vi "SerialFrameProtocol_1_test.vi"() -> ()   [LabVIEW 2015]
uses:
  <vilib>/Instr/_visa.llb/VISA Flush IO Buffer Mask.ctl
  <vilib>/Instr/_visa.llb/VISA Set IO Buffer Mask.ctl
  <vilib>/Instr/_visa.llb/VISA Configure Serial Port (Instr).vi
panel:
  in  "VISA resource name":refnum<visa-resource-name>="COM6"
  out "buffer, NORMAL == read buffer unstuffing, NORMAL":bool
  out "size(s)":i32
  out "size(s)":i32
  out "Receiv Array":u8[](array[numeric])
  out "Send Array":u8[](array[numeric])
  out "Data2 (U16)":u16[](array[numeric])
  out "size(Data2)":i32
  out "size(Data1)":i32
  out "Data1 (I32)":i32[](array[numeric])
  out "B0":cluster{"iVal":i32, "fVal":sgl}
  out "buffer, HEX":string
  out "buffer, NORMAL":string
  out "buffer stuffing, HEX":string
  in  "Clear log":bool
  in  "CA":bool
  out "log":string
  in  "CL":bool
  in  "CZ":bool
  out "VISA Read counter":i32
  out "error IO":errorcluster
  out "VISA Read no error counter":i32
  in  "CN":bool
  in  "CY":bool
  in  "CB":bool
  out "CX Send array == AX read array":bool
  out "read buffer unstuffing, HEX":string
  out "read buffer unstuffing, NORMAL":string
  out "buffer stuffing, NORMAL":string
  out "read buffer RAW, HEX":string
  in  "stop":bool
  out "Counter":i32
  out "read buffer RAW, NORMAL":string="\n"
  in  "CX Send rand array":bool
  # "Serial Frame Protocol Test"
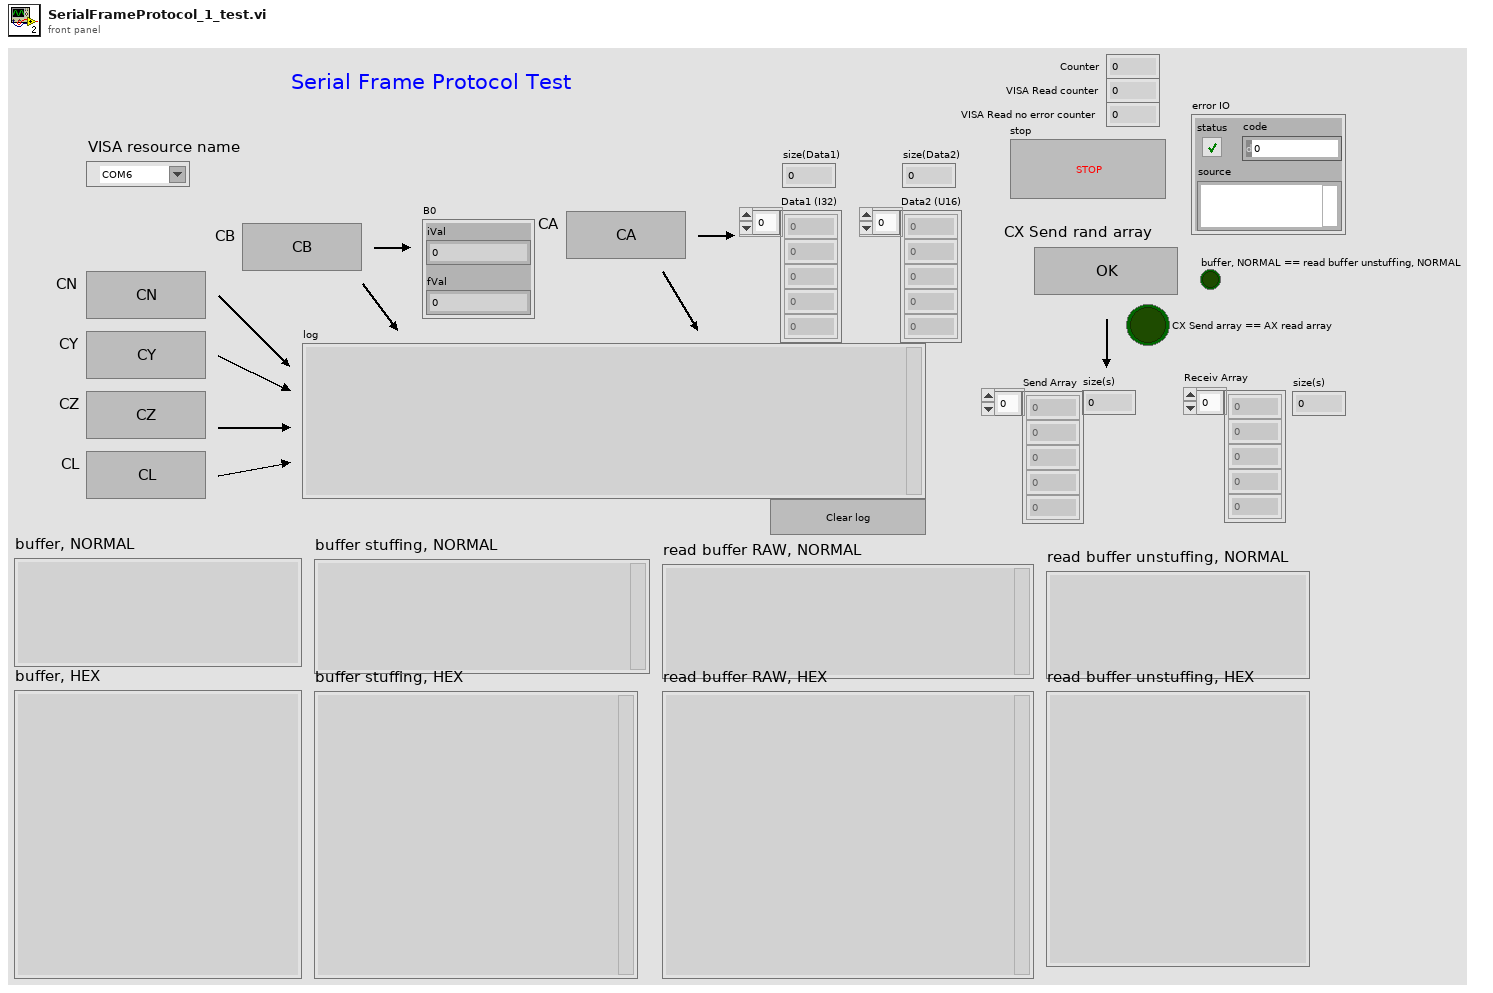
[diagram p1: front panel]
types:
  T1 = typedef "VISA Set IO Buffer Mask.ctl" = u16
  T2 = typedef "VISA Flush IO Buffer Mask.ctl" = u16
  T3 = enum16{"big-endian, network order", "native, host order", "little-endian"}
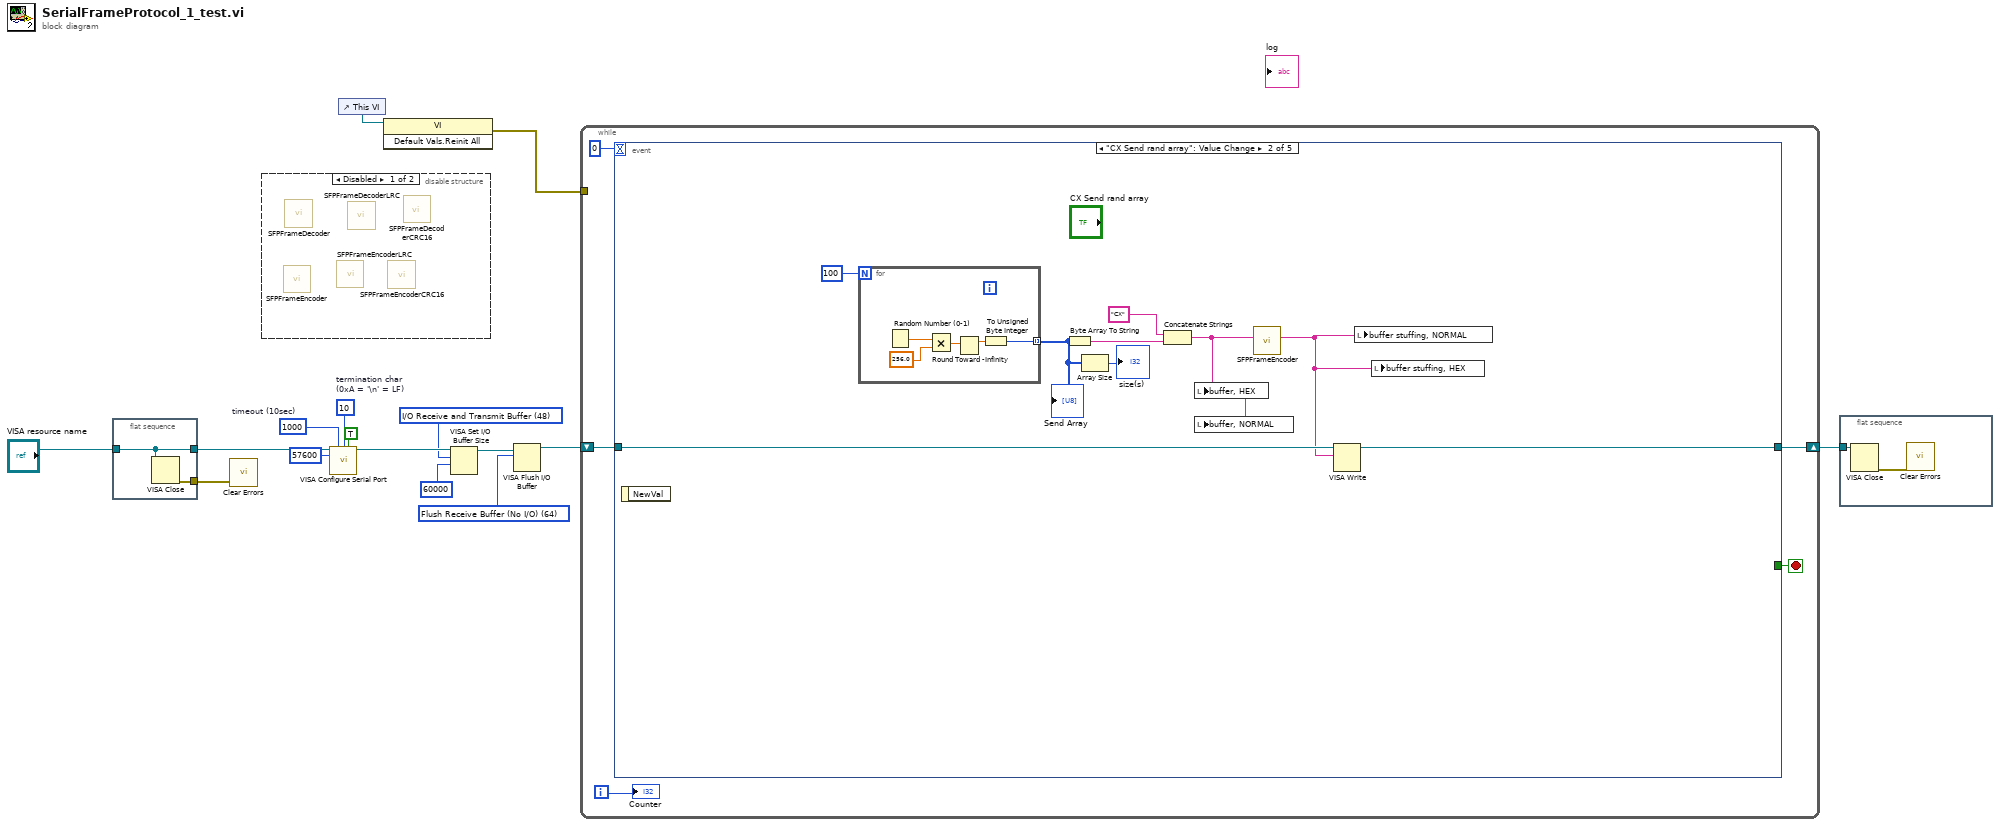
[diagram p0: block diagram]
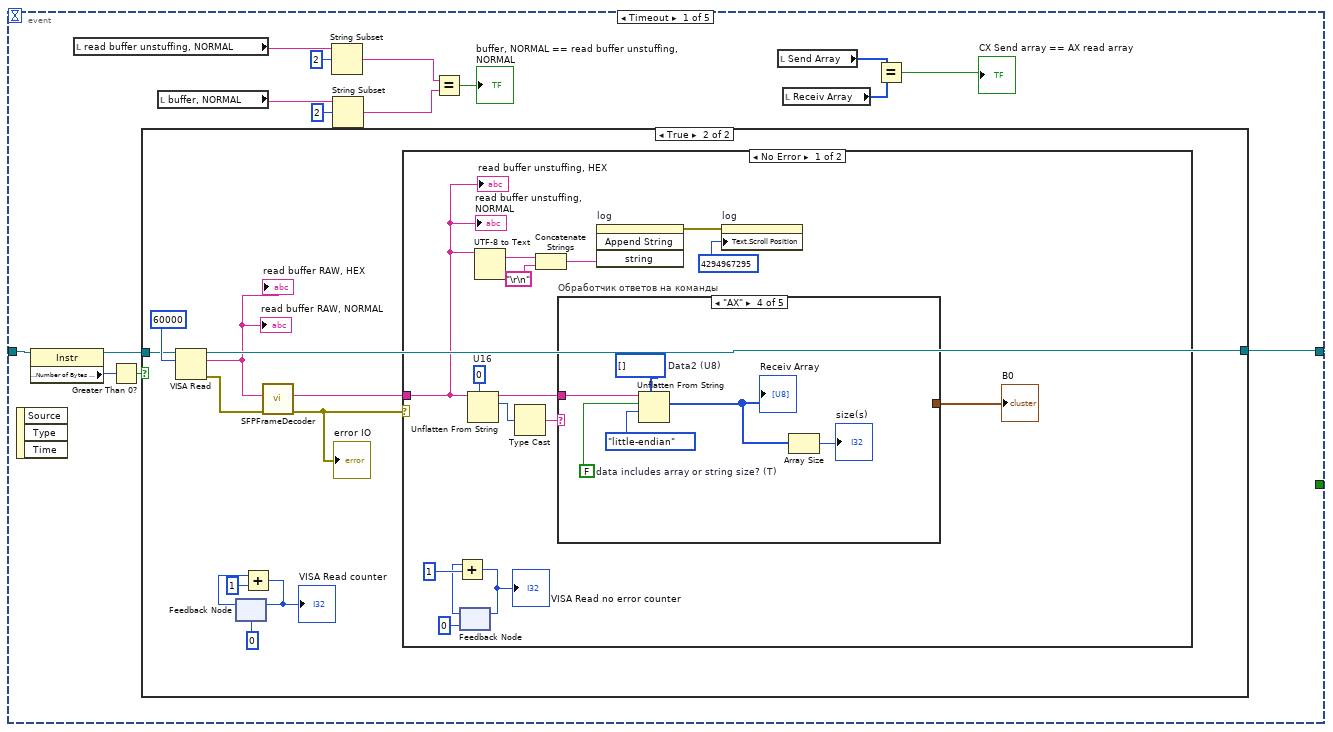
[diagram p2: hidden frame]
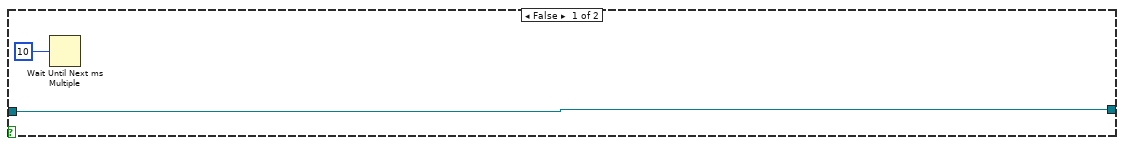
[diagram p3: hidden frame]
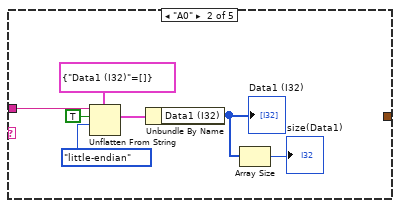
[diagram p5: hidden frame]
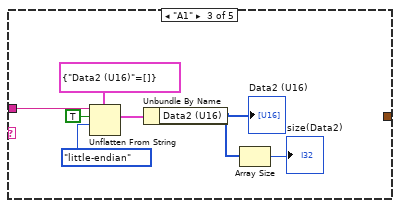
[diagram p6: hidden frame]
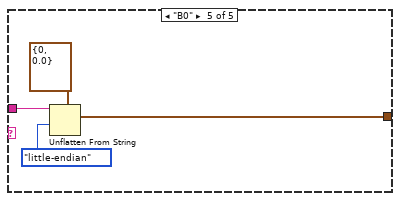
[diagram p7: hidden frame]
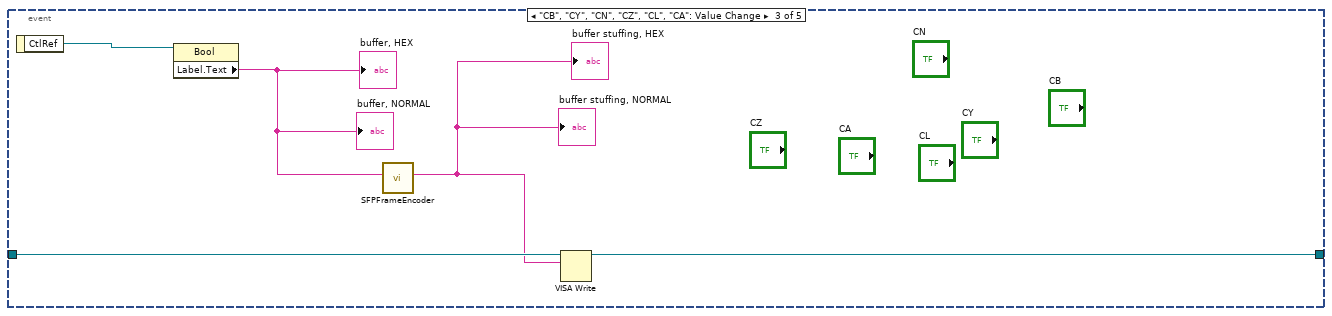
[diagram p9: hidden frame]
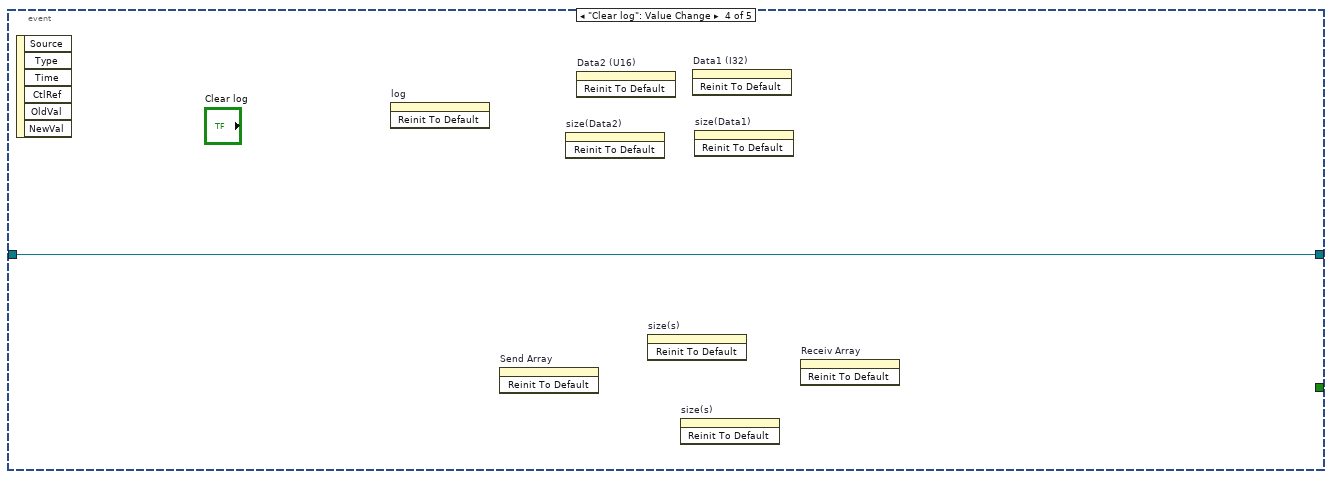
[diagram p10: hidden frame]
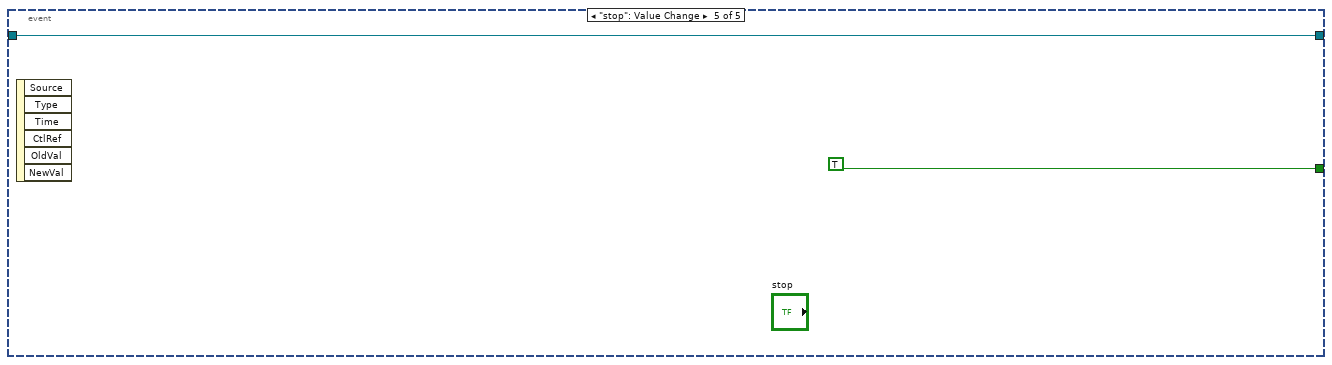
[diagram p11: hidden frame]
diagram:
  w3 = T1 48 items=["I/O Receive Buffer"=16, "I/O Transmit Buffer"=32, "I/O Receive and Transmit Buffer"=48] ("Mask")
  w5 = T2 64 items=["Flush Receive Buffer"=16, "Write Transmit Buffer to Device"=32, "Flush Receive Buffer (No I/O)"=64, "Flush Transmit Buffer"=128] ("Mask")
  w11 = u8 10  # termination char (0xA = '\n' = LF)
  w13 = u32 1000  # timeout (10sec)
  n1 = flat-sequence {
    tunnel: "VISA resource name" -> [w18]
    tunnel: [w18] -> w9
    tunnel: [w17] -> w16
    frame #0 {
      n2 = VISA Close(VISA resource name=w18) -> (error out=w17:errorcluster)  [unwired: 1 in]
    }
  }
  n3 = call <vilib>:"Clear Errors.vi"("error in (no error)"=w16) -> ()  [unwired: 5 in, 2 out]
  n4 = disable-structure shown="Disabled" {
    frame Disabled {
      n5 = call-poly "SFPFrameEncoder.vi"() -> ()  [unwired: 4 in, 2 out]
      n6 = call-poly "SFPFrameDecoder.vi"() -> ()  [unwired: 6 in, 2 out]
      n7 = call "SFPFrameEncoderLRC.vi"() -> ()  [unwired: 4 in, 2 out]
      n8 = call "SFPFrameDecoderLRC.vi"() -> ()  [unwired: 6 in, 2 out]
      n9 = call "SFPFrameEncoderCRC16.vi"() -> ()  [unwired: 4 in, 2 out]
      n10 = call "SFPFrameDecoderCRC16.vi"() -> ()  [unwired: 6 in, 2 out]
    }
    frame Enabled {
    }
  }
  n11 = call-poly "VISA Configure Serial Port"("VISA resource name"=w9, "timeout (10sec)"=w13, "termination char\n(0xA = '\\n' = LF)"=w11, "Enable Termination\nChar (T)"=TRUE ("Enable Termination\nChar (T)"), "baud rate (9600)"=u32 57600) -> ("VISA resource name out"=w8:refnum<visa-resource-name>)  [unwired: 9 in, 1 out]
  n12 = control-ref of="This VI"() -> (w7:refnum<vi>)
  n13 = invoke class="VI" method="Default Vals.Reinit All"(reference=w7) -> (error out=w6:errorcluster)  [unwired: 2 in, 2 out]
  n14 = VISA Set I/O Buffer Size(VISA resource name=w8, mask (16)=w3, size (4096)=u32 60000) -> (VISA resource name out=w4:refnum<visa-resource-name>)  [unwired: 1 in, 1 out]
  n15 = VISA Flush I/O Buffer(VISA resource name=w4, mask (16)=w5) -> (VISA resource name out=w1:refnum<visa-resource-name>)  [unwired: 1 in, 1 out]
  n16 = while {
    shift-right: [w19] -> w14
    shift-left: w1 -> [w20]
    tunnel: w6 -> [_]
    i -> [w21]
    stop <- w22 stop-if-true
    n17 = event shown="[1] \"CX Send rand array\": Value Change" {
      selector: _ -> [_ _ _ _ _]
      dyn-events: _ -> [_ _ _ _ _]
      timeout: 0 -> [_ _ _ _ _]
      tunnel: [_ _ _ _ TRUE] -> w22
      tunnel: w20 -> [w35 w98 w108 w110 w111]
      tunnel: [w34 w97 w107 w110 w111] -> w19
      event Timeout {
        n18 = event-data() -> ()  [unwired: 1 in, 3 out]
        n19 = property class="Instr"(reference=w35) -> (reference out=w36:refnum<visa-resource-name>, "Serial Settings:Number of Bytes at Serial Port"=w37:u32)  [unwired: 1 in, 1 out]
        n20 = local read "read buffer unstuffing, NORMAL"() -> (w32:string)
        n21 = Greater Than 0?(x=w37) -> (x > 0?=w38:bool)
        n22 = case shown="True" w38 {
          tunnel: [w40 w46] -> w34
          tunnel: w36 -> [w40 w45]
          frame False {
            n23 = Wait Until Next ms Multiple(millisecond multiple=u32 10) -> ()  [unwired: 1 out]
          }
          frame True {
            n24 = VISA Read(VISA resource name=w45, byte count=u32 60000) -> (VISA resource name out=w46:refnum<visa-resource-name>, read buffer=w42:string, error out=w44:errorcluster)  [unwired: 1 in, 1 out]
            "read buffer RAW, NORMAL" <- w42
            "read buffer RAW, HEX" <- w42
            n25 = feedback #1(0) -> (w48:i32)
            n26 = Add(x=w48, y=1) -> (x+y=w49:i32)
            "VISA Read counter" <- w49
            n27 = feedback-in #1(w49) -> ()
            n28 = call-poly "SFPFrameDecoder.vi"("error in (no error)"=w44, "Encoded frame"=w42) -> ("error out"=w41:errorcluster, "Decoded data"=w43:string)  [unwired: 4 in]
            "error IO" <- w41
            n29 = case shown="No Error" w41 {
              tunnel: w43 -> [w57 _]
              frame No Error {
                w56 = u16 0  # U16
                n30 = feedback #2(0) -> (w65:i32)
                n31 = Add(x=w65, y=1) -> (x+y=w64:i32)
                "VISA Read no error counter" <- w64
                n32 = feedback-in #2(w64) -> ()
                n33 = Unflatten From String(type=w56, binary string=w57) -> (rest of the binary string=w53:string, value=w54:u16)  [unwired: 3 in, 1 out]
                n34 = UTF-8 to Text(11:w57) -> (3:w58:string)  [unwired: 2 in, 1 out]
                n35 = Type Cast(x=w54) -> (*(type *) &x=w55:string)  [unwired: 1 in]
                n36 = Concatenate Strings(w58, "\r\n") -> (w60:string)
                n37 = case "Обработчик ответов на команды" shown="\"AX\"" w55 {
                  tunnel: w53 -> [_ w71 w78 w85 w88]
                  tunnel: [_ _ _ _ w87] -> w52
                  frame Default {
                    # "Пустой обрабтчик"
                  }
                  frame "A0" {
                    n38 = Unflatten From String(type=cluster{"Data1 (I32)":i32[]} {"Data1 (I32)"=[]}, binary string=w71, data includes array or string size? (T)=TRUE, byte order (0:big-endian, network order)=T3."little-endian") -> (value=w69:cluster{"Data1 (I32)":i32[]})  [unwired: 1 in, 2 out]
                    n39 = Unbundle By Name(w69) -> ("Data1 (I32)"=w68:i32[])
                    "Data1 (I32)" <- w68
                    n40 = Array Size(array=w68) -> (size(s)=→"size(Data1)":i32)
                  }
                  frame "A1" {
                    n41 = Unflatten From String(type=cluster{"Data2 (U16)":u16[]} {"Data2 (U16)"=[]}, binary string=w78, data includes array or string size? (T)=TRUE, byte order (0:big-endian, network order)=T3."little-endian") -> (value=w76:cluster{"Data2 (U16)":u16[]})  [unwired: 1 in, 2 out]
                    n42 = Unbundle By Name(w76) -> ("Data2 (U16)"=w75:u16[])
                    "Data2 (U16)" <- w75
                    n43 = Array Size(array=w75) -> (size(s)=→"size(Data2)":i32)
                  }
                  frame "AX" {
                    w82 = u8[] []  # Data2 (U8)
                    w84 = FALSE  # data includes array or string size? (T)
                    n44 = Unflatten From String(type=w82, binary string=w85, data includes array or string size? (T)=w84, byte order (0:big-endian, network order)=T3."little-endian") -> (value=w81:u8[])  [unwired: 1 in, 2 out]
                    "Receiv Array" <- w81
                    n45 = Array Size(array=w81) -> (size(s)=→"size(s)":i32)
                  }
                  frame "B0" {
                    n46 = Unflatten From String(type=cluster{"iVal":i32, "fVal":sgl} {"iVal"=0, "fVal"=0.0}, binary string=w88, byte order (0:big-endian, network order)=T3."little-endian") -> (value=w87:cluster{"iVal":i32, "fVal":sgl})  [unwired: 2 in, 2 out]
                  }
                }
                "B0" <- w52
                n47 = invoke on="log" class="Str" method="Append String"("string"=w60) -> (error out=w61:errorcluster)  [unwired: 3 in, 3 out]
                n48 = property on="log" class="Str"(error in=w61, "Text.Scroll Position"=u32 4294967295) -> ()  [unwired: 1 in, 2 out]
                "read buffer unstuffing, HEX" <- w57
                "read buffer unstuffing, NORMAL" <- w57
              }
              frame Error {
              }
            }
          }
        }
        n49 = local read "buffer, NORMAL"() -> (w30:string)
        n50 = String Subset(string=w32, offset (0)=2) -> (substring=w29:string)  [unwired: 1 in]
        n51 = String Subset(string=w30, offset (0)=2) -> (substring=w28:string)  [unwired: 1 in]
        n52 = Equal?(x=w29, y=w28) -> (x = y?=→"buffer, NORMAL == read buffer unstuffing, NORMAL":bool)
        n53 = local read "Send Array"() -> (w27:u8[])
        n54 = local read "Receiv Array"() -> (w26:u8[])
        n55 = Equal?(x=w27, y=w26) -> (x = y?=→"CX Send array == AX read array":bool)
      }
      event "CX Send rand array": Value Change {
        n56 = event-data() -> ()  [unwired: 1 in, 1 out]
        n57 = for {
          N: 100 -> [_]
          tunnel: [w100] -> w92 mode=indexing
          n58 = Random Number (0-1)() -> (number: 0 to 1=w104:dbl)
          n59 = Multiply(x=w104, y=256.0) -> (x*y=w102:dbl)
          n60 = Round Toward -Infinity(1:w102) -> (0:w101:dbl)
          n61 = To Unsigned Byte Integer(number=w101) -> (unsigned 8bit integer=w100:u8)
        }
        "Send Array" <- w92
        n62 = Byte Array To String(unsigned byte array=w92) -> (string=w94:string)
        n63 = Array Size(array=w92) -> (size(s)=→"size(s)":i32)
        n64 = Concatenate Strings("CX" ("string"), w94) -> (w93:string)
        n65 = local write "buffer, HEX"(w93) -> ()
        n66 = local write "buffer, NORMAL"(w93) -> ()
        n67 = call-poly "SFPFrameEncoder.vi"("Data"=w93) -> ("Encoded frame"=w95:string)  [unwired: 5 in, 1 out]
        n68 = VISA Write(VISA resource name=w98, write buffer=w95) -> (VISA resource name out=w97:refnum<visa-resource-name>)  [unwired: 1 in, 2 out]
        n69 = local write "buffer stuffing, NORMAL"(w95) -> ()
        n70 = local write "buffer stuffing, HEX"(w95) -> ()
      }
      event "CB", "CY", "CN", "CZ", "CL", "CA": Value Change {
        n71 = event-data() -> ("CtlRef"=w109:refnum<vi>)  [unwired: 1 in]
        n72 = property class="Bool"(reference=w109) -> ("Label.Text"=w105:string)  [unwired: 1 in, 2 out]
        "buffer, NORMAL" <- w105
        "buffer, HEX" <- w105
        n73 = call-poly "SFPFrameEncoder.vi"("Data"=w105) -> ("Encoded frame"=w106:string)  [unwired: 5 in, 1 out]
        "buffer stuffing, HEX" <- w106
        "buffer stuffing, NORMAL" <- w106
        n74 = VISA Write(VISA resource name=w108, write buffer=w106) -> (VISA resource name out=w107:refnum<visa-resource-name>)  [unwired: 1 in, 2 out]
      }
      event "Clear log": Value Change {
        n75 = event-data() -> ()  [unwired: 1 in, 6 out]
        n76 = invoke on="log" class="Str" method="Reinit To Default"() -> ()  [unwired: 3 in, 3 out]
        n77 = invoke on="Send Array" class="Arr (strict)" method="Reinit To Default"() -> ()  [unwired: 3 in, 3 out]
        n78 = invoke on="size(Data2)" class="DigNum (strict)" method="Reinit To Default"() -> ()  [unwired: 3 in, 3 out]
        n79 = invoke on="Data2 (U16)" class="Arr (strict)" method="Reinit To Default"() -> ()  [unwired: 3 in, 3 out]
        n80 = invoke on="size(s)" class="DigNum (strict)" method="Reinit To Default"() -> ()  [unwired: 3 in, 3 out]
        n81 = invoke on="size(s)" class="DigNum (strict)" method="Reinit To Default"() -> ()  [unwired: 3 in, 3 out]
        n82 = invoke on="Data1 (I32)" class="Arr (strict)" method="Reinit To Default"() -> ()  [unwired: 3 in, 3 out]
        n83 = invoke on="size(Data1)" class="DigNum (strict)" method="Reinit To Default"() -> ()  [unwired: 3 in, 3 out]
        n84 = invoke on="Receiv Array" class="Arr (strict)" method="Reinit To Default"() -> ()  [unwired: 3 in, 3 out]
      }
      event "stop": Value Change {
        n85 = event-data() -> ()  [unwired: 1 in, 6 out]
      }
    }
    "Counter" <- w21
  }
  n86 = flat-sequence {
    tunnel: w14 -> [w114]
    frame #0 {
      n87 = VISA Close(VISA resource name=w114) -> (error out=w113:errorcluster)  [unwired: 1 in]
      n88 = call <vilib>:"Clear Errors.vi"("error in (no error)"=w113) -> ()  [unwired: 5 in, 2 out]
    }
  }
